vi "Final Product.vi"() -> ()   [LabVIEW 2020]
panel:
  in  "STOP":bool
  in  "?":bool
  # "WELCOME TO THE WORLD\nOF GESTURES !!!"
  # "WELCOME TO THE WORLD\nOF GESTURES !!!"
  # "PRESS ENTER TO CONTINUE..."
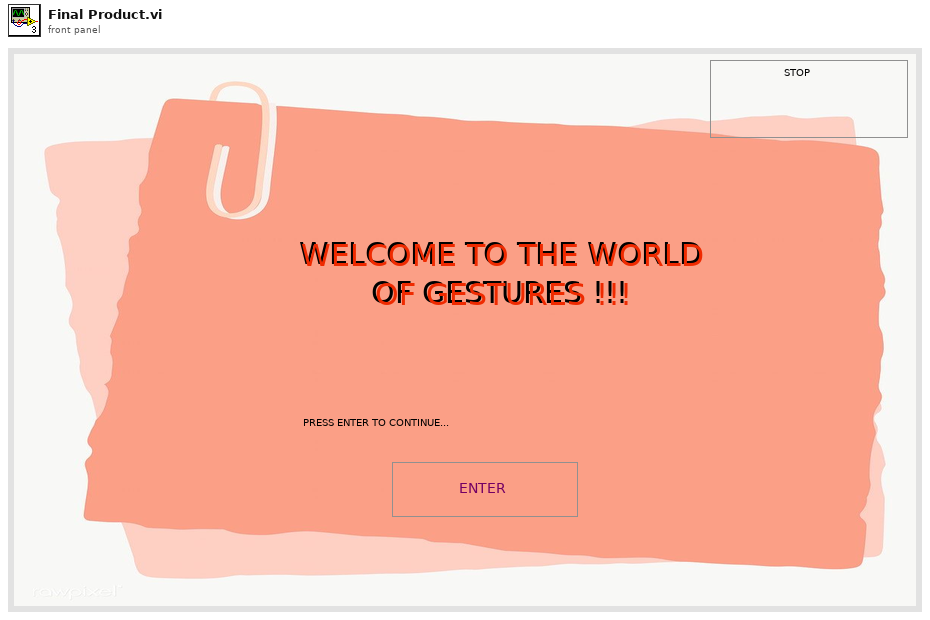
[diagram p1: front panel]
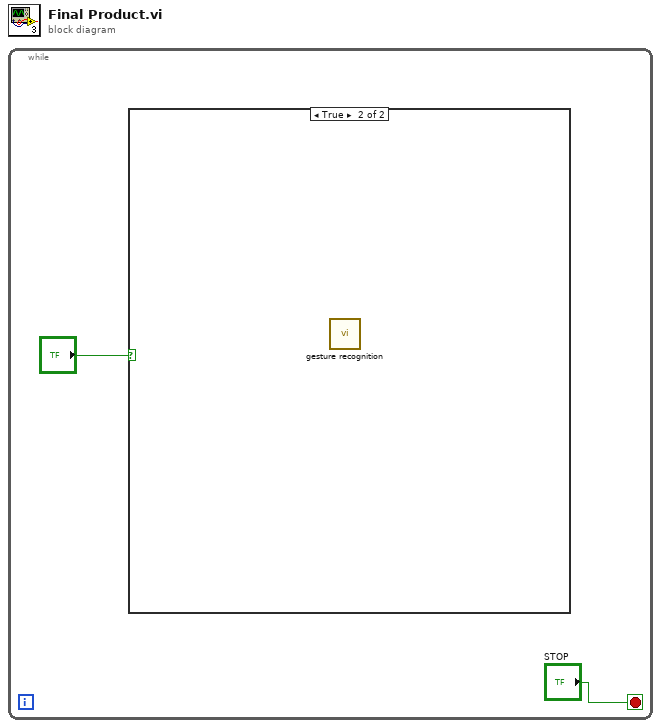
[diagram p0: block diagram]
diagram:
  n1 = while {
    stop <- "STOP" stop-if-true
    n2 = case shown="True" "?" {
      frame False {
      }
      frame True {
        n3 = call "gesture recognition.vi"() -> ()  [unwired: 12 in]
      }
    }
  }
